vi "Philosofers.vi"() -> ()   [LabVIEW 2015]
uses:
  SINGLE_CHOP_Separator_string.ctl
panel:
  in  "Algorithm":u8(knob) scale=0.0..2.0
  in  "Eating attempts.":i32=100
  in  "Maximum think time":u32=160
  in  "Maximum eat time":u32=100
  in  "How many philosofers ?":i32=24 min=2 step=1
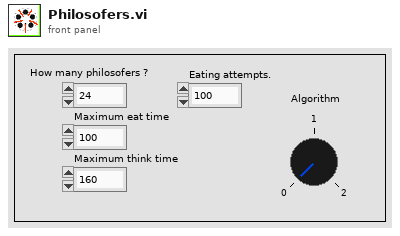
[diagram p1: front panel]
types:
  T1 = typedef "SINGLE_CHOP_Separator_string.ctl" = string
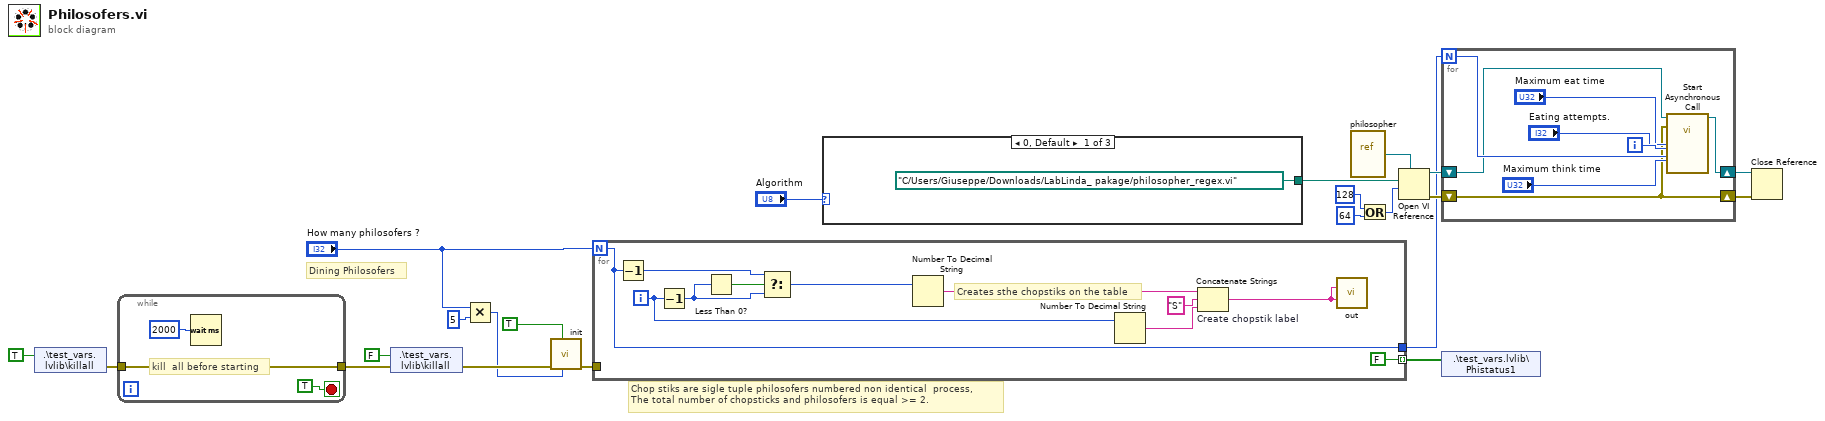
[diagram p0: block diagram]
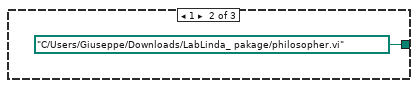
[diagram p2: hidden frame]
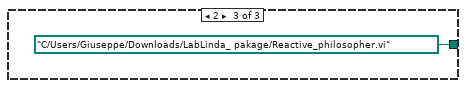
[diagram p3: hidden frame]
diagram:
  # "Chop stiks are sigle tuple philosofers numbered non identical  process,\nThe total number of chopsticks and philosofers is equal >= 2."
  # "Dining Philosofers"
  n1 = shared-variable ".\\test_vars.lvlib\\killall"(TRUE ("killall")) -> (error out=w5:errorcluster)  [unwired: 1 in]
  n2 = while {
    tunnel: w5 -> [w23]
    tunnel: [w23] -> w4
    stop <- TRUE stop-if-true
    # "kill  all before starting"
    n3 = Wait (ms)(milliseconds to wait=u32 2000) -> ()  [unwired: 1 out]
  }
  n4 = shared-variable ".\\test_vars.lvlib\\killall"(FALSE ("killall"), error in=w4) -> (error out=w19:errorcluster)
  n5 = Multiply(x="How many philosofers ?", y=5) -> (x*y=w7:i32)
  n6 = call "init.vi"("Space size"=w7, "Cleaneup"=TRUE ("Cleneup"), "error in (no error)"=w19) -> ("error out"=w21:errorcluster)  [unwired: 8 in]
  n7 = for {
    N: "How many philosofers ?" -> [w27]
    tunnel: w21 -> [_]
    tunnel: [w27] -> w3
    tunnel: [FALSE] -> w18 mode=indexing
    i -> [w34]
    # "Creates sthe chopstiks on the table"
    n8 = Decrement(x=w27) -> (x-1=w30:i32)
    n9 = Decrement(x=w34) -> (x-1=w35:i32)
    n10 = Less Than 0?(x=w35) -> (x < 0?=w36:bool)
    n11 = Select(t=w30, s=w36, f=w35) -> (s? t:f=w33:i32)
    n12 = Number To Decimal String(number=w33) -> (decimal integer string=w31:string)  [unwired: 1 in]
    n13 = Number To Decimal String(number=w34) -> (decimal integer string=w29:string)  [unwired: 1 in]
    n14 = Concatenate Strings "Create chopstik label"(w31, T1 "S", w29) -> (w32:string)
    n15 = call "out.vi"("IN VARIANT"=w32, "Name in"=w32) -> ()  [unwired: 12 in, 2 out]
  }
  n16 = case shown="0, Default" "Algorithm" {
    tunnel: [path "C:/Users/Giuseppe/Downloads/LabLinda_ pakage/philosopher_regex.vi" ("vi path") path "C:/Users/Giuseppe/Downloads/LabLinda_ pakage/philosopher.vi" ("vi path") path "C:/Users/Giuseppe/Downloads/LabLinda_ pakage/Reactive_philosopher.vi" ("vi path")] -> w1
    frame 0, Default {
    }
    frame 1 {
    }
    frame 2 {
    }
  }
  n17 = vi-ref "philosopher.vi"() -> (w17:refnum<vi>)
  n18 = Or(x=128 ("options"), y=64) -> (x .or. y?=w10:i32)
  n19 = Open VI Reference(type specifier VI Refnum (for type only)=w17, vi path=w1, options=w10) -> (vi reference=w16:refnum<vi>, error out=w14:errorcluster)  [unwired: 3 in]
  n20 = for {
    N: w3 -> [w46]
    shift-right: [w40] -> w13
    shift-left: w14 -> [w40]
    shift-right: [w42] -> w15
    shift-left: w16 -> [w41]
    i -> [w47]
    n21 = call-by-ref "Start Asynchronous Call"(reference=w41, error in=w40, "Maximum attempts"="Eating attempts.", "Maximum think time"="Maximum think time", "Maximum eat time"="Maximum eat time", "total"=w46, "Ph id"=w47) -> (reference out=w42:refnum<vi>)  [unwired: 7 in, 1 out]
  }
  n22 = shared-variable ".\\test_vars.lvlib\\Phistatus1"(w18) -> ()  [unwired: 1 in, 1 out]
  n23 = Close Reference(reference=w15, error in (no error)=w13) -> ()  [unwired: 1 out]
